vi "NextObject.vi"(8 "error in (no error)":errorcluster, 11 "CompositeIterator":refnum<class "CompositeIterator.lvclass">) -> (0 "error out":errorcluster, 2 "BrowerComponent":refnum<class "BrowerComponent.lvclass">, 3 "CompositeIterator out":refnum<class "CompositeIterator.lvclass">)   [LabVIEW 2015, in "CompositeIterator.lvclass"]
uses:
  CompositeIterator.lvclass
  BrowerComponent/BrowerComponent/BrowerComponent.lvclass
  BrowerComponent/BrowerComposite/BrowerComposite.lvclass
  CompositeIterator.lvclass/CompositeIterator.ctl
  ArrayIterator/ArrayIterator.lvclass
  Interface/Iterator.lvclass
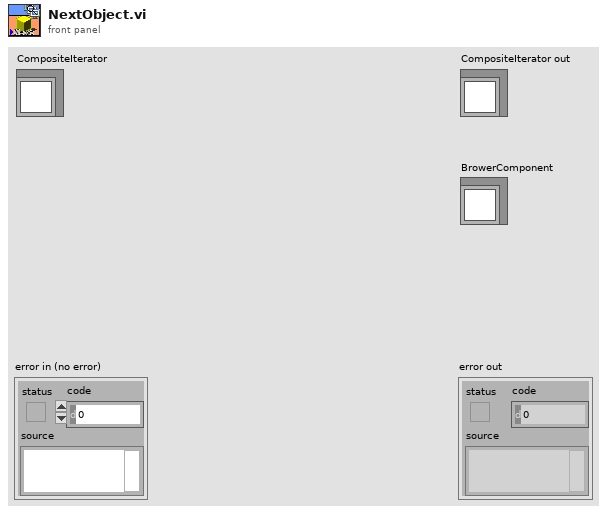
[diagram p1: front panel]
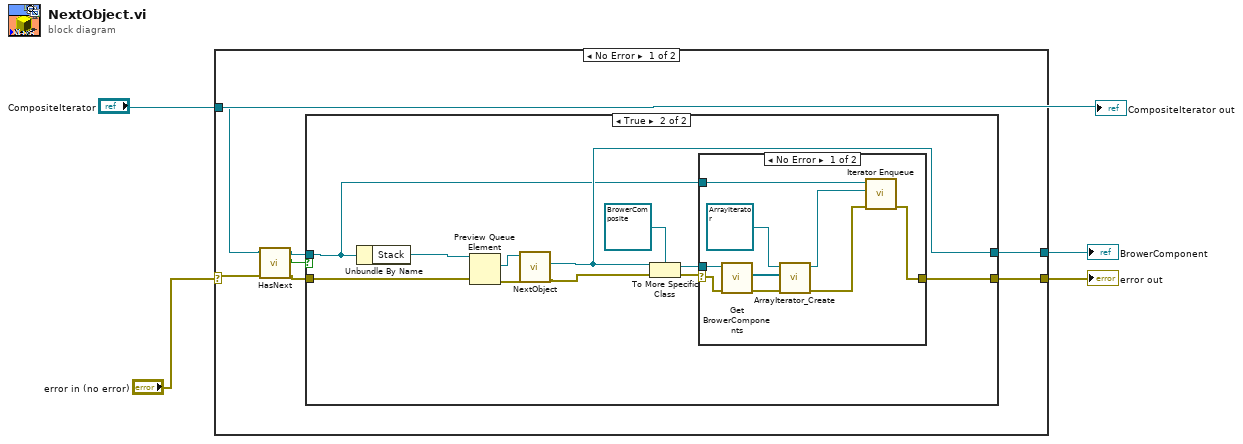
[diagram p0: block diagram]
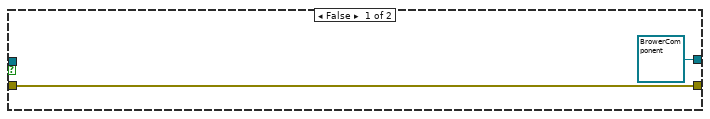
[diagram p2: hidden frame]
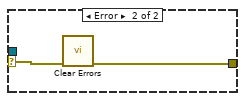
[diagram p3: hidden frame]
diagram:
  n1 = case shown="No Error" "error in (no error)" {
    selector: "error in (no error)" -> [w8 w36]
    tunnel: "CompositeIterator" -> [w9 _]
    tunnel: [w11 w36] -> w4
    tunnel: [w10 _] -> w3
    frame No Error {
      n2 = call-dynamic "HasNext.vi"("error in (no error)"=w8, "CompositeIterator"=w9) -> ("error out"=w5:errorcluster, "HasNext?(False)"=w7:bool, "CompositeIterator Out"=w6:refnum<class "CompositeIterator.lvclass">)  [unwired: 7 in]
      n3 = case shown="True" w7 {
        tunnel: w6 -> [_ w14]
        tunnel: w5 -> [w13 w19]
        tunnel: [refnum<class "BrowerComponent.lvclass"> refnum ("BrowerComponent") w16] -> w10
        tunnel: [w13 w21] -> w11
        frame False {
        }
        frame True {
          n4 = Unbundle By Name(w14) -> ("Stack"=w20:refnum<queue>)
          n5 = Preview Queue Element(queue=w20, error in (no error)=w19) -> (element=w18:refnum<class "Iterator.lvclass">, error out=w17:errorcluster)  [unwired: 1 in, 2 out]
          n6 = call-dynamic "NextObject.vi"("error in (no error)"=w17, "Iterator"=w18) -> ("error out"=w15:errorcluster, "BrowerComponent"=w16:refnum<class "BrowerComponent.lvclass">)  [unwired: 7 in, 1 out]
          n7 = To More Specific Class(target class=refnum<class "BrowerComposite.lvclass"> refnum ("BrowerComposite"), reference=w16, error in=w15) -> (specific class reference=w22:refnum<class "BrowerComposite.lvclass">, error out=w23:errorcluster)
          n8 = case shown="No Error" w23 {
            selector: w23 -> [w32 w35]
            tunnel: w14 -> [w28 _]
            tunnel: w22 -> [w33 _]
            tunnel: [w25 w34] -> w21
            frame No Error {
              n9 = call "Get BrowerComponents.vi"("error in (no error)"=w32, "BrowerComposite in"=w33) -> ("error out"=w30:errorcluster, "BrowerComponents"=w31:refnum<class "BrowerComponent.lvclass">[])  [unwired: 7 in, 1 out]
              n10 = call "ArrayIterator_Create.vi"("error in (no error)"=w30, "BrowerComponents"=w31, "reference in"=refnum<class "ArrayIterator.lvclass"> refnum) -> ("error out"=w26:errorcluster, "reference out"=w27:refnum<class "ArrayIterator.lvclass">)  [unwired: 7 in]
              n11 = call-dynamic "Iterator Enqueue.vi"("error in (no error)"=w26, "Iterator"=w27, "CompositeIterator in"=w28) -> ("error out"=w25:errorcluster)  [unwired: 7 in, 1 out]
            }
            frame Error {
              n12 = call <vilib>:"Clear Errors.vi"("error in (no error)"=w35) -> ("error out"=w34:errorcluster)  [unwired: 5 in, 1 out]
            }
          }
        }
      }
    }
    frame Error {
    }
  }
  "error out" <- w4
  "BrowerComponent" <- w3
  "CompositeIterator out" <- "CompositeIterator"
